vi "PLC Write Find.vi"(7 "Data1 In":T1(c390), 8 "error in (no error)":errorcluster caption="Error In", 9 "Data In":string, 10 "Data":T2, 11 "PLC.PLC":refnum<k5>) -> (0 "error out":errorcluster caption="Error Out")   [LabVIEW 2020]
uses:
  Global/Data Global/SDQ Data Type.ctl
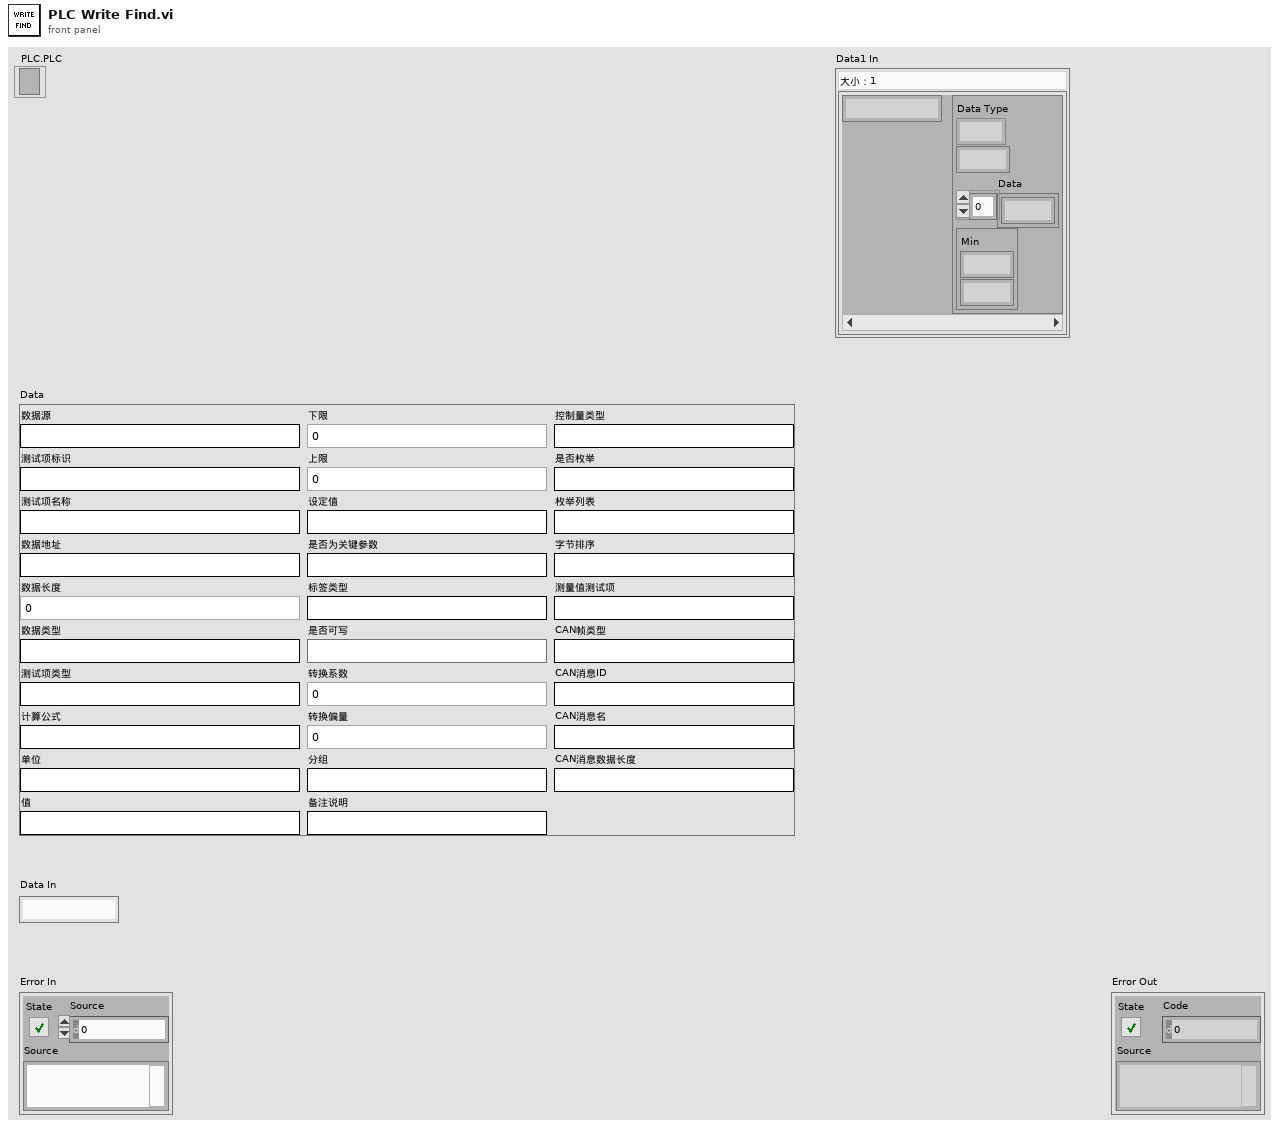
[diagram p1: front panel]
types:
  T1 = map{string, cluster{"Data Type":enum16{"I", "Q", "M", "D", "Count", "Timer"}, u16, "Data":u8[], cluster{"Min":u16, u16}}}
  T2 = typedef "SDQ Data Type.ctl" = cluster{"CAN Length":string, "CAN Name":string, "CAN ID":string, "CAN Type":string, "Test Item":string, "Byte Order":string, "Instruction":string, "Control Type":string, "Group":string, "Offset":dbl, "Coefficient":dbl, "Write Enable":bool, "Lable Type":string, "Key?":string, "Set Value":string, "Upper":dbl, "Lower":dbl, "Unit":string, "Formula":string, "Test Item Type":string, "Length":i32, "Address":string, "Name":string, "Identifier":string, "Data Type":string, "Enumerate?":string, "Enumerate List":string, "Data":string, "Source":string}
  T3 = cluster{"Data Type":enum16{"I", "Q", "M", "D", "Count", "Timer"}, u16, "Data":u8[], cluster{"Min":u16, u16}}
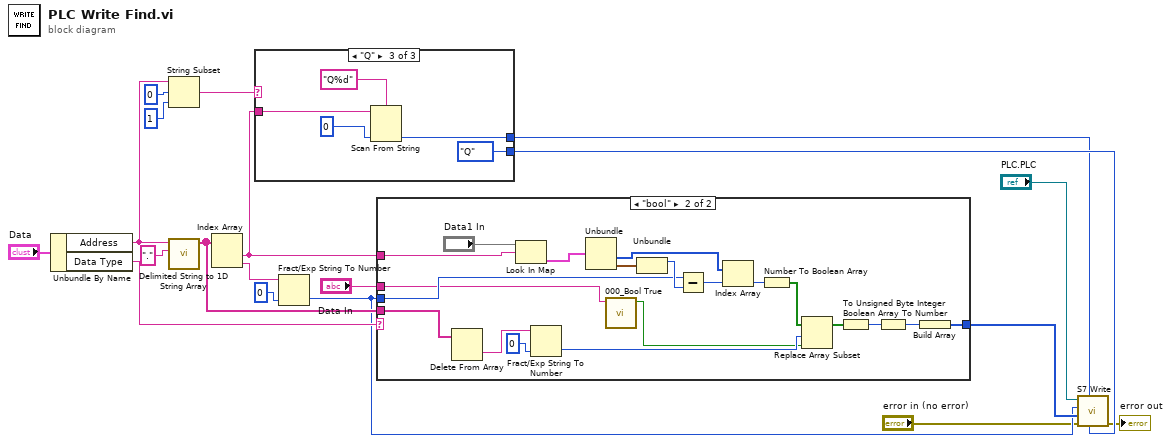
[diagram p0: block diagram]
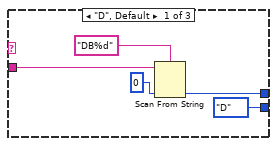
[diagram p2: hidden frame]
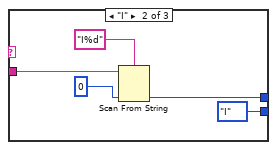
[diagram p3: hidden frame]
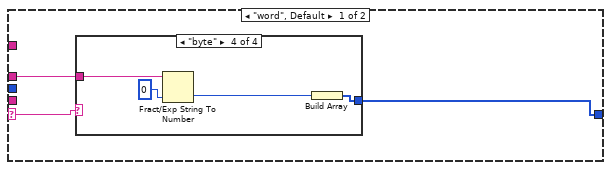
[diagram p4: hidden frame]
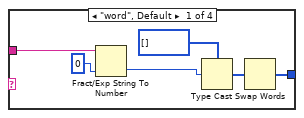
[diagram p5: hidden frame]
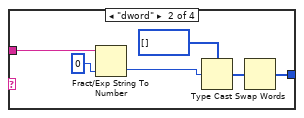
[diagram p6: hidden frame]
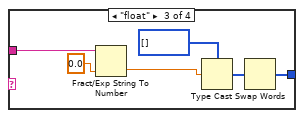
[diagram p7: hidden frame]
diagram:
  n1 = Unbundle By Name("Data") -> ("Address"=w10:string, "Data Type"=w15:string)
  n2 = String Subset(string=w10, offset (0)=0 ("偏移量(0)"), length (rest)=1 ("长度（剩余）")) -> (substring=w14:string)
  n3 = call <vilib>:"Delimited String to 1D String Array.vi"("delimiter"=".", "delimited string"=w10) -> ("string array"=w7:string[])  [unwired: 9 in]
  n4 = Index Array(array=w7) -> (element #1=w6:string, element #2=w8:string)  [unwired: 2 in]
  n5 = case shown="\"Q\"" w14 {
    tunnel: [enum16{"I", "Q", "M", "D", "Count", "Timer"}."D" ("Data Type") enum16{"I", "Q", "M", "D", "Count", "Timer"}."I" ("Data Type") enum16{"I", "Q", "M", "D", "Count", "Timer"}."Q" ("Data Type")] -> w18
    tunnel: w6 -> [w22 w26 w31]
    tunnel: [w21 w27 w32] -> w16
    frame "D", Default {
      n6 = Scan From String(format string="DB%d" ("格式字符串"), input string=w22, default 1=u16 0 ("默认值 1")) -> (output 1=w21:u16)  [unwired: 2 in, 3 out]
    }
    frame "I" {
      n7 = Scan From String(format string="I%d" ("格式字符串"), input string=w26, default 1=u16 0 ("默认值 1")) -> (output 1=w27:u16)  [unwired: 2 in, 3 out]
    }
    frame "Q" {
      n8 = Scan From String(format string="Q%d" ("格式字符串"), input string=w31, default 1=u16 0 ("默认值 1")) -> (output 1=w32:u16)  [unwired: 2 in, 3 out]
    }
  }
  n9 = Fract/Exp String To Number(string=w8, default (0 dbl)=u16 0 ("默认(0 DBL)")) -> (number=w3:u16)  [unwired: 2 in, 1 out]
  n10 = case shown="\"bool\"" w15 {
    selector: w15 -> [w37 _]
    tunnel: [w36 w71] -> w19
    tunnel: w7 -> [_ w70]
    tunnel: w6 -> [_ w69]
    tunnel: "Data In" -> [w35 w61]
    tunnel: w3 -> [_ w63]
    frame "word", Default {
      n11 = case shown="\"byte\"" w37 {
        tunnel: [w38 w47 w53 w59] -> w36
        tunnel: w35 -> [w41 w45 w51 w57]
        frame "word", Default {
          n12 = Fract/Exp String To Number(string=w41, default (0 dbl)=u16 0) -> (number=w40:u16)  [unwired: 2 in, 1 out]
          n13 = Type Cast(type=u8[] [], x=w40) -> (*(type *) &x=w39:u8[])
          n14 = Swap Words(1:w39) -> (0:w38:u8[])
        }
        frame "dword" {
          n15 = Fract/Exp String To Number(string=w45, default (0 dbl)=u32 0) -> (number=w44:u32)  [unwired: 2 in, 1 out]
          n16 = Type Cast(type=u8[] [], x=w44) -> (*(type *) &x=w48:u8[])
          n17 = Swap Words(1:w48) -> (0:w47:u8[])
        }
        frame "float" {
          n18 = Fract/Exp String To Number(string=w51, default (0 dbl)=sgl 0.0 ("默认(0 DBL)")) -> (number=w50:sgl)  [unwired: 2 in, 1 out]
          n19 = Type Cast(type=u8[] [], x=w50) -> (*(type *) &x=w54:u8[])
          n20 = Swap Words(1:w54) -> (0:w53:u8[])
        }
        frame "byte" {
          n21 = Fract/Exp String To Number(string=w57, default (0 dbl)=u8 0) -> (number=w56:u8)  [unwired: 2 in, 1 out]
          n22 = Build Array(w56) -> (w59:u8[])
        }
      }
    }
    frame "bool" {
      n23 = Delete From Array(array=w70) -> (deleted portion=w79:string)  [unwired: 2 in, 1 out]
      n24 = Look In Map(map="Data1 In", key=w69) -> (value=w68:T3)  [unwired: 1 in, 1 out]
      n25 = Fract/Exp String To Number(string=w79, default (0 dbl)=0 ("默认(0 DBL)")) -> (number=w75:i32)  [unwired: 2 in, 1 out]
      n26 = Unbundle(w68) -> ("Data"=w66:u8[], w67:cluster{"Min":u16, u16})  [unwired: 2 out]
      n27 = call "000_Bool True.vi"("Bool String"=w61) -> ("True"=w60:bool)  [unwired: 8 in, 2 out]
      n28 = Unbundle(w67) -> ("Min"=w65:u16)  [unwired: 1 out]
      n29 = Subtract(x=w63, y=w65) -> (x-y=w64:u16)
      n30 = Index Array(array=w66, index=w64) -> (element=w77:u8)
      n31 = Number To Boolean Array(number=w77) -> (Boolean array=w76:bool[])
      n32 = Replace Array Subset(array=w76, new element=w60, index=w75) -> (w74:bool[])
      n33 = Boolean Array To Number(Boolean array=w74) -> (number=w73:u32)
      n34 = To Unsigned Byte Integer(number=w73) -> (unsigned 8bit integer=w72:u8)
      n35 = Build Array(w72) -> (w71:u8[])
    }
  }
  n36 = call "S7 Write.vi"("Data Type"=w18, "DB block"=w16, "Error In"="error in (no error)", "Write Byte"=w19, "Start Address"=w3, "TCP In"="PLC.PLC") -> ("Error out"=→"error out":errorcluster)  [unwired: 4 in, 1 out]
